vi "Generate Table Data.vi"(8 "error in (no error)":errorcluster, 10 "Entity Type":T1, 11 "Coffee Shop in":refnum<class "Coffee Shop.lvclass">) -> (0 "error out":errorcluster, 3 "Coffee Shop out":refnum<class "Coffee Shop.lvclass">)   [LabVIEW 2023, in "Coffee Shop.lvlib" / "Coffee Shop.lvclass"]
doc: "Extracts the details of a particular entity type (baristas, cashiers, or customers), reformats it, and sends it to UI for display."
uses:
  Coffee Shop.lvclass
  Entity Types.ctl
  Coffee Shop.lvclass/Coffee Shop.ctl
  Table Data.ctl
  Entity Table/Entity Table.lvclass
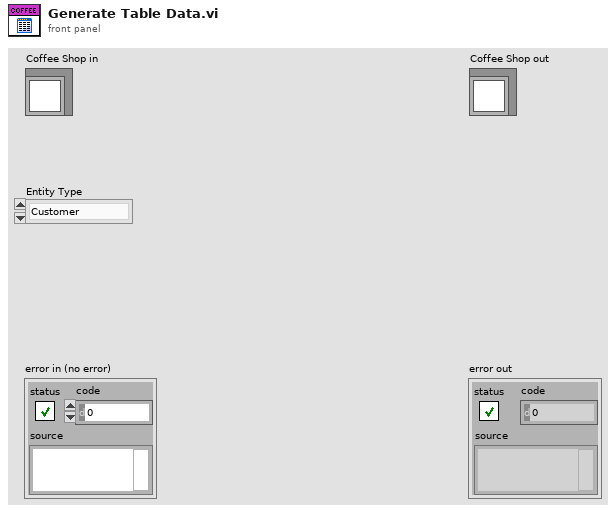
[diagram p1: front panel]
types:
  T1 = typedef "Coffee Shop.lvlib/Coffee Shop.lvclass/Entity Types.ctl" = enum16{"Customer", "Cashier", "Barista"}
  T2 = typedef "Coffee Shop.lvlib/Coffee Shop.lvclass/Table Data.ctl" = cluster{"Entity Type":T1, "Item Names":string[][]}
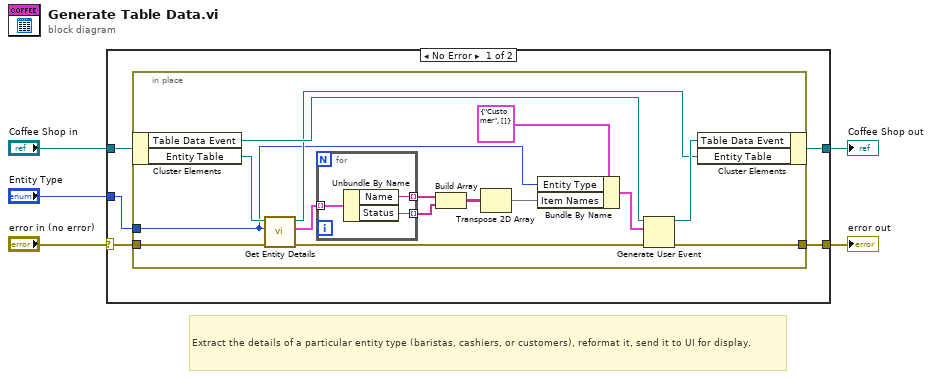
[diagram p0: block diagram]
diagram:
  # "Extract the details of a particular entity type (baristas, cashiers, or customers), reformat it, send it to UI for display."
  n1 = case shown="No Error" "error in (no error)" {
    selector: "error in (no error)" -> [w6 w30]
    tunnel: [w10 w30] -> w4
    tunnel: [w7 w29] -> w2
    tunnel: "Coffee Shop in" -> [w8 w29]
    tunnel: "Entity Type" -> [w9 _]
    frame No Error {
      n2 = in-place "In Place Element Structure" {
        in-place-border: [w24] -> w10
        in-place-border: w9 -> [w11]
        in-place-border: w6 -> [w17]
        n3 = in-place-cluster #1 ("Unbundle / Bundle Elements")(w8) -> ("Table Data Event"=w20:refnum<user-event>, "Entity Table"=w18:refnum<class "Entity Table.lvclass">)
        n4 = call-dynamic "Get Entity Details.vi"("error in (no error)"=w17, "Entity Type"=w11, "Entity Table in"=w18) -> ("error out"=w16:errorcluster, "Entity Details"=w14:cluster{"Name":string, "Status":string}[], "Entity Table out"=w15:refnum<class "Entity Table.lvclass">)  [unwired: 6 in]
        n5 = for {
          tunnel: w14 -> [w28] mode=indexing
          tunnel: [w27] -> w13 mode=indexing
          tunnel: [w26] -> w12 mode=indexing
          n6 = Unbundle By Name(w28) -> ("Name"=w27:string, "Status"=w26:string)
        }
        n7 = Build Array(w13, w12) -> (w22:string[][])
        n8 = Transpose 2D Array(2D array=w22) -> (transposed array=w21:string[][])
        n9 = Bundle By Name(cluster=T2 {"Entity Type"=enum."Customer", "Item Names"=[]} ("Table Data"), "Entity Type"=w11, "Item Names"=w21) -> (w25:T2)
        n10 = Generate User Event(user event=w20, event data cluster=w25, error in=w16) -> (user event out=w19:refnum<user-event>, error out=w24:errorcluster)  [unwired: 1 in]
        n11 = in-place-cluster #1 ("Unbundle / Bundle Elements")("Table Data Event"=w19, "Entity Table"=w15) -> (w7:refnum<class "Coffee Shop.lvclass">)
      }
    }
    frame Error {
    }
  }
  "error out" <- w4
  "Coffee Shop out" <- w2
